vi "ROS close.vi"(8 "DataIn":T1) -> (0 "error out":errorcluster, 2 "Opcode":u8, 3 "Data":string)   [LabVIEW 2015]
uses:
  <vilib>/MediaMongrels Ltd/WebSockets/WebSockets/WebSockets.lvlib
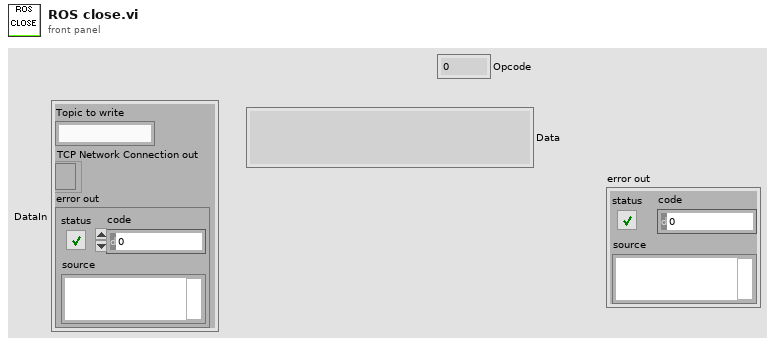
[diagram p1: front panel]
types:
  T1 = cluster{"Topic to write":string, "TCP Network Connection out":refnum<k5>, "error out":errorcluster}
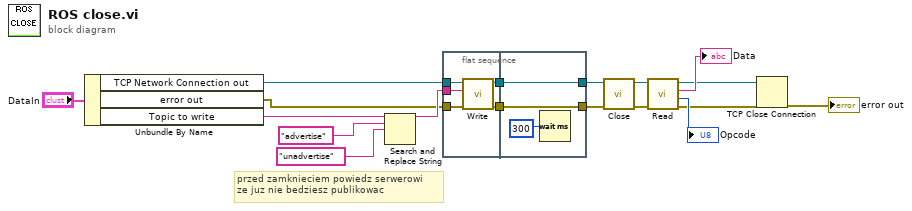
[diagram p0: block diagram]
diagram:
  # "przed zamknieciem powiedz serwerowi\nze juz nie bedziesz publikowac"
  n1 = Unbundle By Name("DataIn") -> ("TCP Network Connection out"=w3:refnum<k5>, "error out"=w2:errorcluster, "Topic to write"=w1:string)
  n2 = Search and Replace String(input string=w1, search string="advertise", replace string="unadvertise" ("search string")) -> (result string=w8:string)  [unwired: 5 in, 3 out]
  n3 = flat-sequence {
    tunnel: w3 -> [w23]
    tunnel: w2 -> [w22]
    tunnel: w8 -> [w21]
    tunnel: [w20] -> w18
    tunnel: [w19] -> w17
    tunnel: [w25] -> w7
    tunnel: [w26] -> w6
    tunnel: w18 -> [w26]
    tunnel: w17 -> [w25]
    frame #0 {
      n4 = call <vilib>:"Write.vi"("error in (no error)"=w22, "Data"=w21, "WebSocket Connection in"=w23) -> ("error out"=w19:errorcluster, "WebSocket Connection out"=w20:refnum<k5>)  [unwired: 7 in]
    }
    frame #1 {
      n5 = Wait (ms)(milliseconds to wait=u32 300) -> ()  [unwired: 1 out]
    }
  }
  n6 = call <vilib>:"Close.vi"("error in (no error)"=w7, "WebSocket Connection in"=w6) -> ("error out"=w12:errorcluster, "WebSocket Connection in"=w11:refnum<k5>)  [unwired: 8 in]
  n7 = call <vilib>:"Read.vi"("error in (no error)"=w12, "WebSocket Connection in"=w11) -> ("error out"=w13:errorcluster, "Opcode"=→"Opcode":u8, "Data"=→"Data":string, "WebSocket Connection out"=w14:refnum<k5>)  [unwired: 6 in]
  n8 = TCP Close Connection(connection ID=w14, error in (no error)=w13) -> (error out=→"error out":errorcluster)  [unwired: 1 in, 1 out]
